vi "Update Loaded Plugins by Reference.vi"(8 "error in (no error)":errorcluster, 10 "Plugin Summary Info":T1[](array[typedef]), 11 "Loaded Plugins ref in":refnum<vi>) -> (0 "error out":errorcluster, 3 "Loaded Plugins ref out":refnum<vi>)   [LabVIEW 2021, in "CIF_Manager_UI.lvclass"]
uses:
  CIF_Manager_UI.lvclass
  <vilib>/CIF Foundation/CIF Core/CIFUI/Typedef/Plugin Summary.ctl
  <vilib>/CIF Foundation/CIF Core/CIFCore/Common/Typedef/Version Simple.ctl
  <vilib>/CIF Foundation/CIF Core/CIFCore/Common/CIFCoreCommon.lvlib
  <vilib>/CIF Foundation/CIF Core/CIFUI/CIF_UI.lvclass
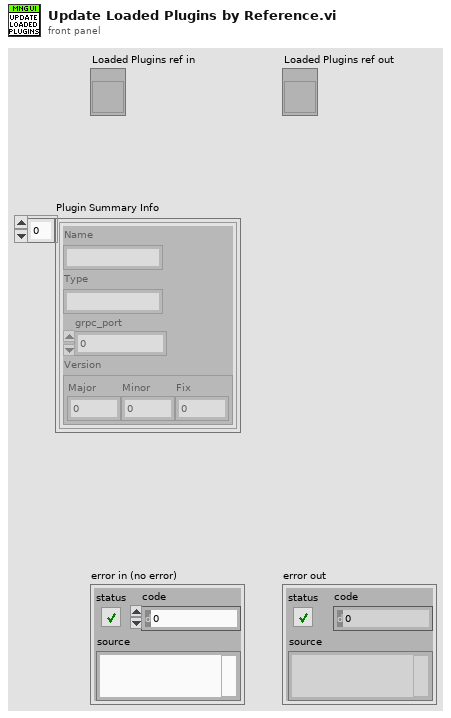
[diagram p1: front panel]
types:
  T1 = typedef "CIF_UI.lvclass/Plugin Summary.ctl" = cluster{"Name":string, "Type":string, "grpc_port":i32, "Version":T2}
  T2 = typedef "CIFCoreCommon.lvlib/Version Simple.ctl" = cluster{"Major":i32, "Minor":i32, "Fix":i32}
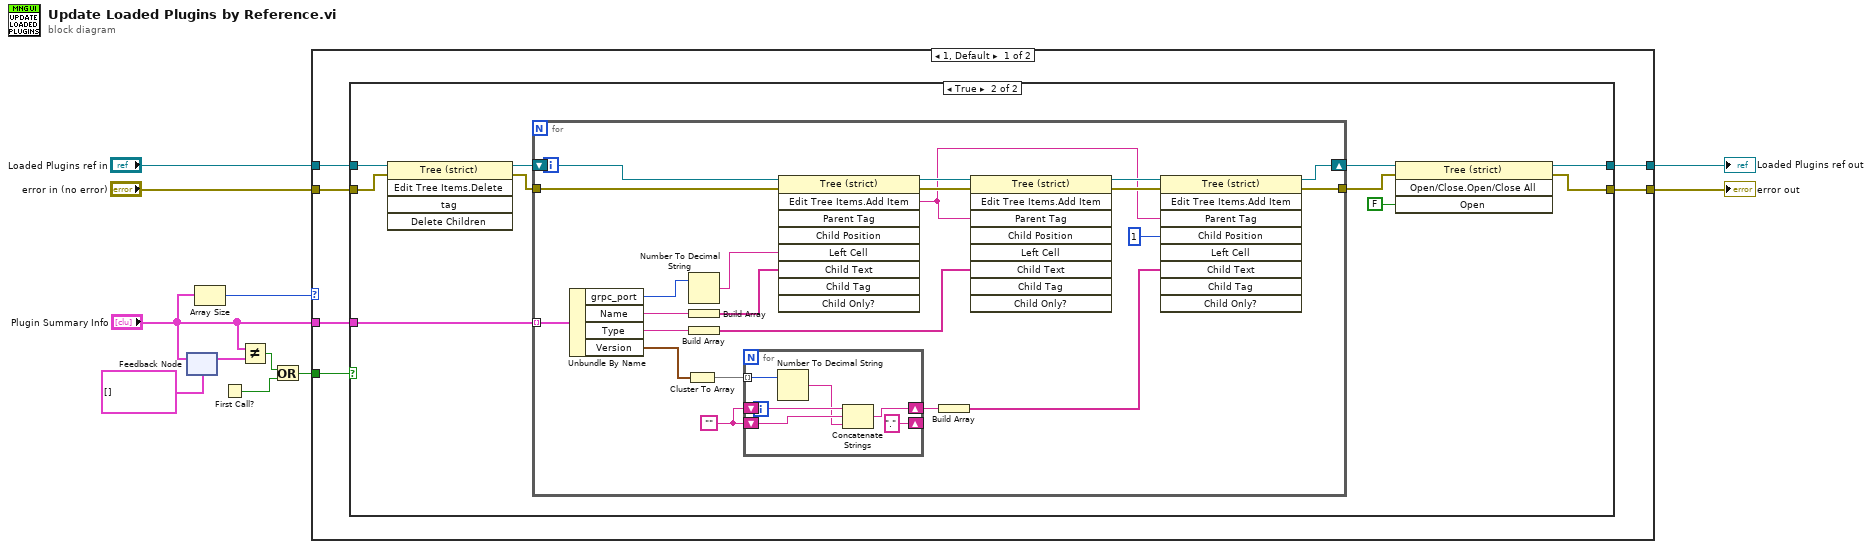
[diagram p0: block diagram]
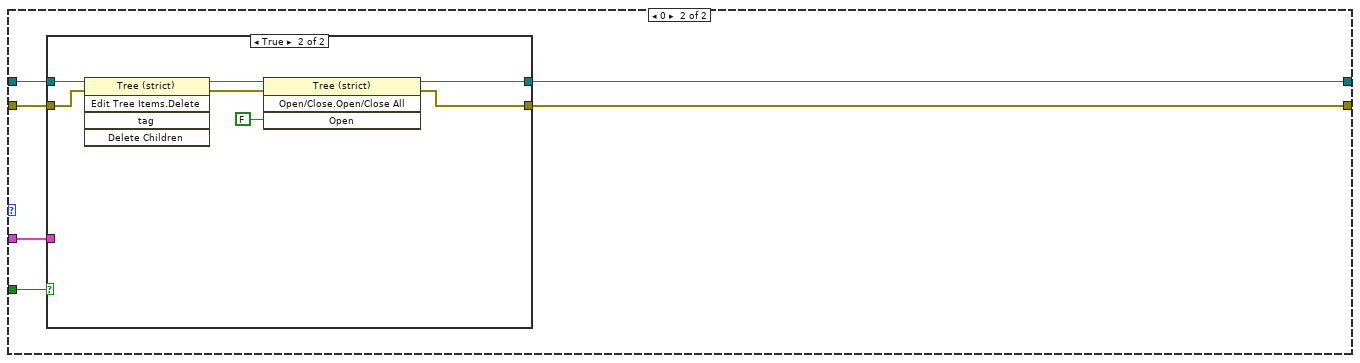
[diagram p3: hidden frame]
diagram:
  n1 = feedback #1(T1[] [] ("Sorted Plugin Info")) -> (w5:T1[])
  n2 = feedback-in #1("Plugin Summary Info") -> ()
  n3 = Array Size(array="Plugin Summary Info") -> (size(s)=w4:i32)
  n4 = First Call?() -> (First Call?: T/F=w2:bool)
  n5 = Not Equal?(x="Plugin Summary Info", y=w5) -> (x != y?=w3:bool)
  n6 = Or(x=w3, y=w2) -> (x .or. y?=w1:bool)
  n7 = case shown="1, Default" w4 {
    tunnel: "error in (no error)" -> [w17 w63]
    tunnel: [w16 w62] -> w10
    tunnel: [w15 w61] -> w9
    tunnel: "Loaded Plugins ref in" -> [w14 w60]
    tunnel: w1 -> [w13 w59]
    tunnel: "Plugin Summary Info" -> [w12 w58]
    frame 1, Default {
      n8 = case shown="True" w13 {
        tunnel: w17 -> [w18 w24]
        tunnel: [w18 w23] -> w16
        tunnel: [w19 w22] -> w15
        tunnel: w14 -> [w19 w21]
        tunnel: w12 -> [_ w20]
        frame False {
        }
        frame True {
          n9 = invoke class="Tree (strict)" method="Edit Tree Items.Delete"(reference=w21, error in=w24) -> (reference out=w28:refnum<vi>, error out=w29:errorcluster)  [unwired: 3 in, 3 out]
          n10 = for {
            tunnel: w29 -> [w34]
            tunnel: [w51] -> w26
            shift-right: [w48] -> w27
            shift-left: w28 -> [w35]
            tunnel: w20 -> [w36] mode=indexing
            w49 = ""
            n11 = Unbundle By Name(w36) -> ("grpc_port"=w37:i32, "Name"=w30:string, "Type"=w41:string, "Version"=w38:T2)
            n12 = Cluster To Array(cluster=w38) -> (array=w50:i32[])
            n13 = Number To Decimal String(number=w37) -> (decimal integer string=w42:string)  [unwired: 1 in]
            n14 = Build Array(w30) -> (w31:string[])
            n15 = Build Array(w41) -> (w33:string[])
            n16 = for {
              tunnel: w50 -> [w52] mode=indexing
              shift-right: ["."] -> _
              shift-left: w49 -> [w56]
              shift-right: [w54] -> w40
              shift-left: w49 -> [w57]
              n17 = Number To Decimal String(number=w52) -> (decimal integer string=w55:string)  [unwired: 1 in]
              n18 = Concatenate Strings(w57, w56, w55) -> (w54:string)
            }
            n19 = invoke class="Tree (strict)" method="Edit Tree Items.Add Item"(reference=w35, error in=w34, "Left Cell"=w42, "Child Text"=w31) -> (reference out=w47:refnum<vi>, error out=w46:errorcluster, "Edit Tree Items:Add Item"=w32:string)  [unwired: 5 in, 6 out]
            n20 = Build Array(w40) -> (w39:string[])
            n21 = invoke class="Tree (strict)" method="Edit Tree Items.Add Item"(reference=w47, error in=w46, "Parent Tag"=w32, "Child Text"=w33) -> (reference out=w45:refnum<vi>, error out=w44:errorcluster)  [unwired: 5 in, 7 out]
            n22 = invoke class="Tree (strict)" method="Edit Tree Items.Add Item"(reference=w45, error in=w44, "Parent Tag"=w32, "Child Position"=1, "Child Text"=w39) -> (reference out=w48:refnum<vi>, error out=w51:errorcluster)  [unwired: 4 in, 7 out]
          }
          n23 = invoke class="Tree (strict)" method="Open/Close.Open/Close All"(reference=w27, error in=w26, "Open"=FALSE ("Open?")) -> (reference out=w22:refnum<vi>, error out=w23:errorcluster)  [unwired: 1 in, 2 out]
        }
      }
    }
    frame 0 {
      n24 = case shown="True" w59 {
        tunnel: w63 -> [w64 w71]
        tunnel: [w64 w70] -> w62
        tunnel: [w65 w69] -> w61
        tunnel: w60 -> [w65 w68]
        tunnel: w58 -> [_ _]
        frame False {
        }
        frame True {
          n25 = invoke class="Tree (strict)" method="Edit Tree Items.Delete"(reference=w68, error in=w71) -> (reference out=w67:refnum<vi>, error out=w66:errorcluster)  [unwired: 3 in, 3 out]
          n26 = invoke class="Tree (strict)" method="Open/Close.Open/Close All"(reference=w67, error in=w66, "Open"=FALSE ("Open?")) -> (reference out=w69:refnum<vi>, error out=w70:errorcluster)  [unwired: 1 in, 2 out]
        }
      }
    }
  }
  "Loaded Plugins ref out" <- w9
  "error out" <- w10
